vi "Test Process Log Finished Lifecycle State.vi"(8 "error in (no error)":errorcluster, 11 "Process Test In":refnum<class "Process Dev Test.lvclass">) -> (0 "error out":errorcluster, 3 "Process Test Out":refnum<class "Process Dev Test.lvclass">)   [LabVIEW 2020, in "Process Dev Test.lvclass"]
uses:
  Process Dev Test.lvclass
  Process Dev Test.lvclass/Process Dev Test.ctl
  source/Framework/Process/Process.lvclass
  source/Framework Test Suite/Mock Log Handler/Mock Log Handler.lvclass
  63cd48a4-71ab-406d-8512-4a07cc0c0a64.vi
  C:/Git/astemes-triarc-framework/source/Framework/Base/Base.lvclass
  C:/Git/astemes-triarc-framework/source/Framework Test Suite/Mock Log Handler/Mock Log Handler.lvclass
  C:/Git/astemes-triarc-framework/source/Framework/Logging/Logging.lvclass
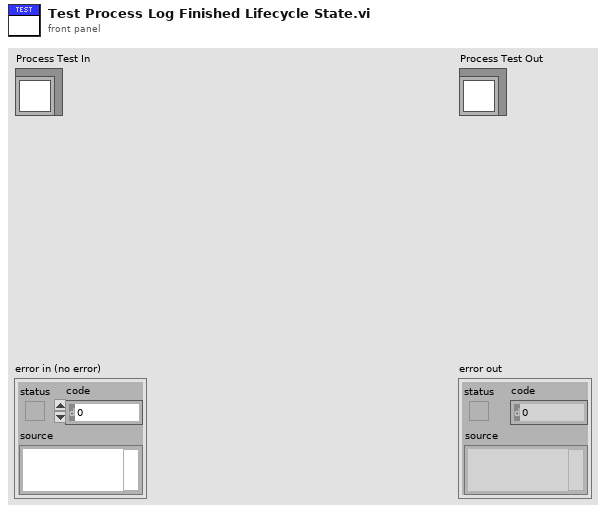
[diagram p1: front panel]
types:
  T1 = typedef "Mock Log Handler.lvclass/Log Entry.ctl" = cluster{"Level":string, "Source":string, "Message":string}
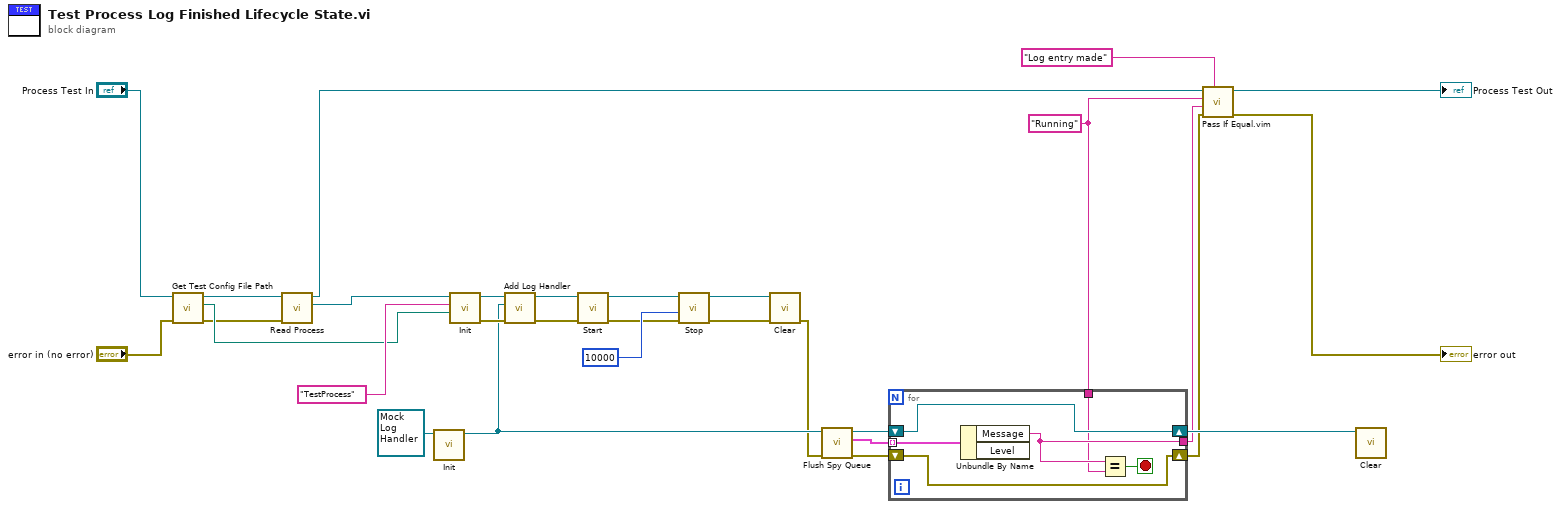
[diagram p0: block diagram]
diagram:
  w1 = "Running"
  n1 = call "Get Test Config File Path.vi"("error in (no error)"="error in (no error)", "Process Test In"="Process Test In") -> ("error out"=w18:errorcluster, "Test config path"=w21:path, "Process Test Out"=w20:refnum<class "Process Dev Test.lvclass">)  [unwired: 7 in]
  n2 = call "Read Process.vi"("error in (no error)"=w18, "Process Test in"=w20) -> ("Process.lvclass"=w19:refnum<class "Process.lvclass">, "Process Test out"=w16:refnum<class "Process Dev Test.lvclass">)  [unwired: 7 in, 1 out]
  n3 = call-dynamic "Init.vi"("Mock Log Handler In"=refnum<class "Mock Log Handler.lvclass"> refnum) -> ("Mock Log Handler Out"=w10:refnum<class "Mock Log Handler.lvclass">)  [unwired: 9 in, 1 out]
  n4 = call-dynamic "Init.vi"("Config File Path"=w21, "Name"="TestProcess", "Process In"=w19) -> ("error out"=w30:errorcluster, "Process Out"=w14:refnum<class "Process.lvclass">)  [unwired: 7 in]
  n5 = call "Add Log Handler.vi"("error in (no error)"=w30, "Log Handler"=w10, "Process In"=w14) -> ("error out"=w24:errorcluster, "Process Out"=w29:refnum<class "Process.lvclass">)  [unwired: 7 in]
  n6 = call "Start.vi"("error in (no error)"=w24, "Process In"=w29) -> ("error out"=w7:errorcluster, "Process Out"=w28:refnum<class "Process.lvclass">)  [unwired: 7 in, 1 out]
  n7 = call "Stop.vi"("error in (no error)"=w7, "timeout in ms (-1)"=10000, "Process In"=w28) -> ("error out"=w5:errorcluster, "Process Out"=w27:refnum<class "Process.lvclass">)  [unwired: 6 in, 1 out]
  n8 = call-dynamic "Clear.vi"("error in (no error)"=w5, "Process In"=w27) -> ("error out"=w4:errorcluster)  [unwired: 9 in]
  n9 = call "Flush Spy Queue.vi"("error in (no error)"=w4, "Mock Log Handler in"=w10) -> ("error out"=w3:errorcluster, "remaining elements"=w2:T1[], "Mock Log Handler out"=w9:refnum<class "Mock Log Handler.lvclass">)  [unwired: 7 in]
  n10 = for {
    shift-right: [w36] -> w12
    shift-left: w9 -> [w36]
    shift-right: [w35] -> w8
    shift-left: w3 -> [w35]
    tunnel: [w34] -> w11
    tunnel: w2 -> [w33] mode=indexing
    tunnel: w1 -> [w31]
    stop <- w32 stop-if-true
    n11 = Unbundle By Name(w33) -> ("Message"=w34:string)  [unwired: 1 out]
    n12 = Equal?(x=w34, y=w31) -> (x = y?=w32:bool)
  }
  n13 = call "Pass If Equal.vim"("Description"="Log entry made", "error in (no error)"=w8, "Actual"=w11, "Expected"=w1, "LUnit Test Case In"=w16) -> ("error out"=→"error out":errorcluster, "LUnit Test Case Out"=→"Process Test Out":refnum<class "Process Dev Test.lvclass">)  [unwired: 5 in]
  n14 = call-dynamic "Clear.vi"("Mock Log Handler In"=w12) -> ()  [unwired: 10 in, 1 out]
